vi "jojo_0822_copy.vi"() -> ()   [LabVIEW 2021]
uses:
  <vilib>/numeric/Random Number (Range) U64.vi
  <vilib>/numeric/sub_Random U32.vi
panel:
  out "Mixed Signal Graph 10":T1(graph)
  out "Mixed Signal Graph 9":T2(graph)
  out "Mixed Signal Graph 8":cluster{"Present (s)":dbl, "number":u64}[](graph)
  out "Mixed Signal Graph 7":cluster{"Present (s)":dbl, "number":u64}[](graph)
  out "Mixed Signal Graph 6":cluster{"Present (s)":dbl, "number":u64}[](graph)
  in  "Press to open Sub VI":bool
  in  "Update, Create, or Index File":string(combo)
  in  "File Name (include extension)":string
  out "error out":errorcluster
  out "Mixed Signal Graph 1":cluster{"Present (s)":dbl, "number":u64}[](graph)
  out "Mixed Signal Graph 2":cluster{"Present (s)":dbl, "number":u64}[](graph)
  out "Mixed Signal Graph 3":cluster{"Present (s)":dbl, "number":u64}[](graph)
  out "Mixed Signal Graph 5":T1(graph)
  out "Mixed Signal Graph 4":T2(graph)
  out "Elapsed Time (s)":dbl format="%<%H:%M:%S\n%y/%m/%d>T"
  out "millisecond timer value":u32
  in  "stop":bool
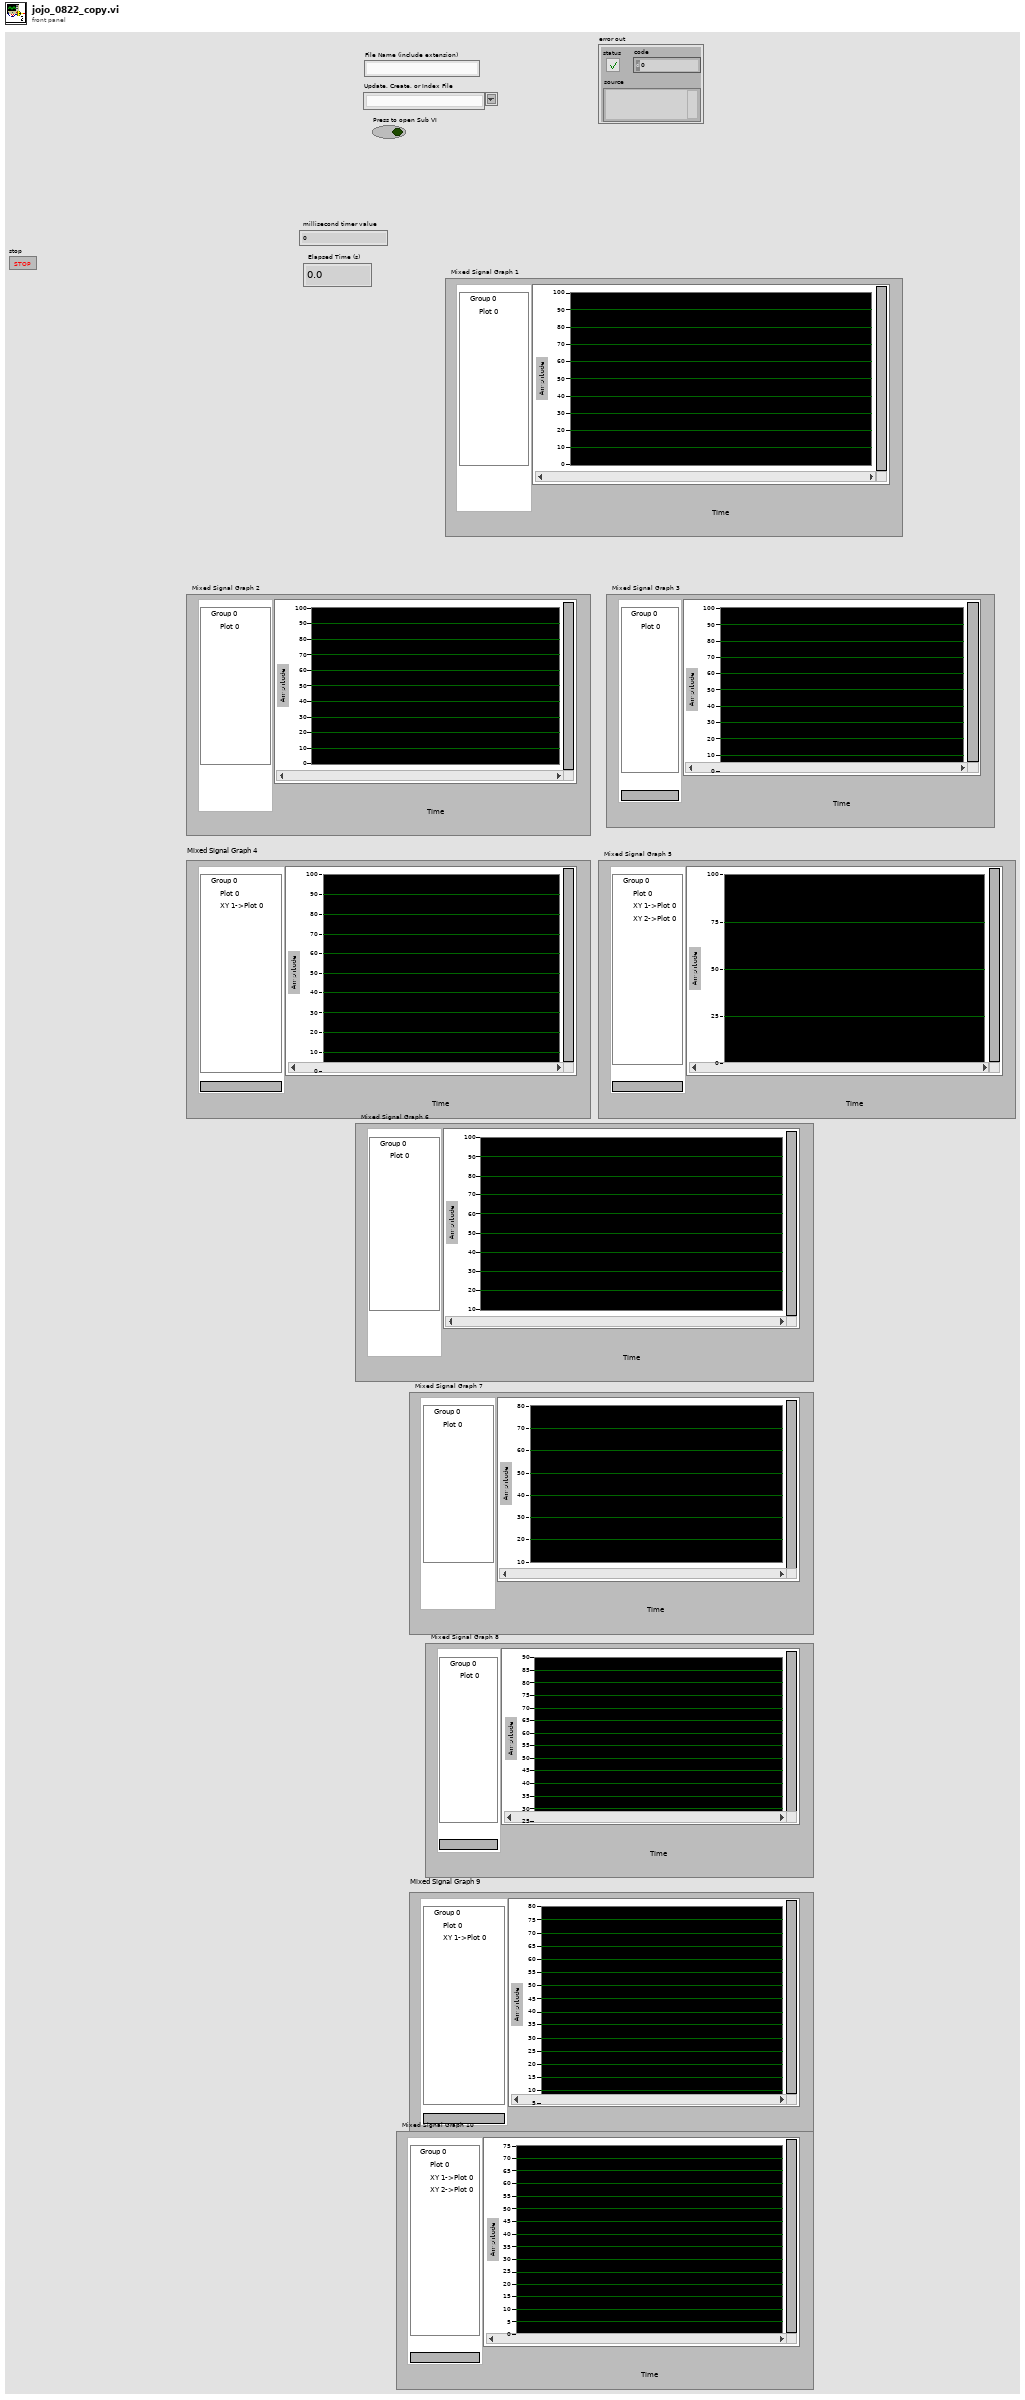
[diagram p1: front panel]
types:
  T1 = cluster{cluster{"Present (s)":dbl, "number":u64}[], cluster{"Present (s)":dbl, "number":u64}[], cluster{"Present (s)":dbl, "number":u64}[]}
  T2 = cluster{cluster{"Present (s)":dbl, "number":u64}[], cluster{"Present (s)":dbl, "number":u64}[]}
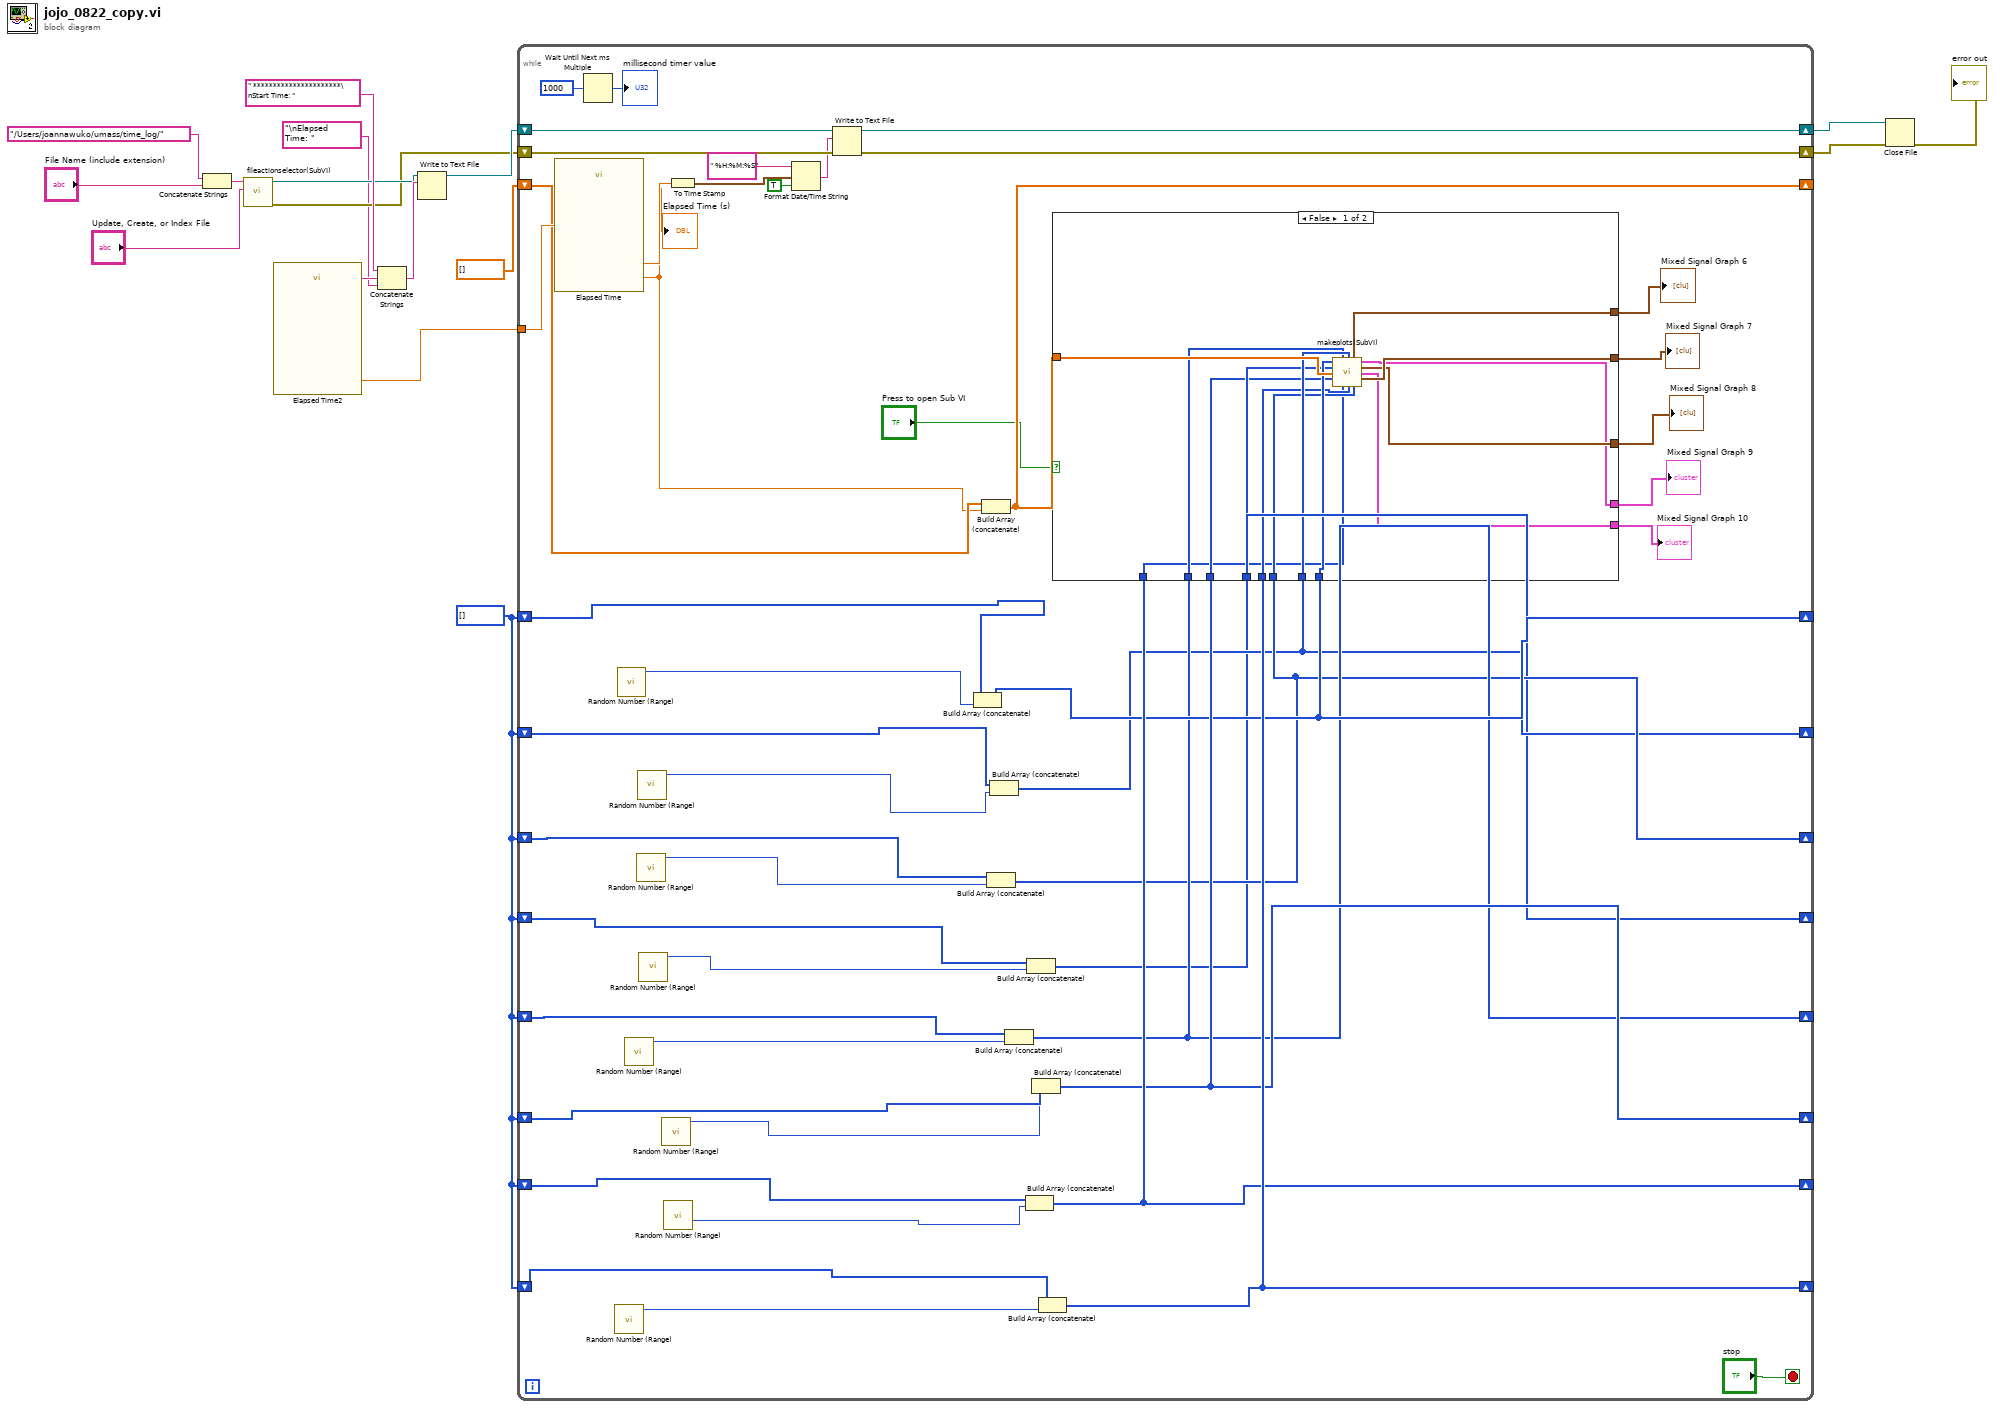
[diagram p0: block diagram]
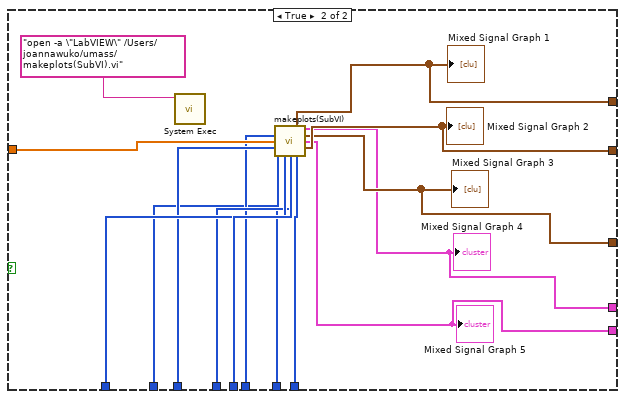
[diagram p2: hidden frame]
diagram:
  w15 = u64[] []
  n1 = Concatenate Strings("/Users/joannawuko/umass/time_log/" ("string"), "File Name (include extension)") -> (w3:string)
  n2 = call "fileactionselector(SubVI).vi"("Choose Update, Create, or Index File"="Update, Create, or Index File", "String"=w3) -> ("error out"=w4:errorcluster, "Byte Stream File out"=w5:refnum<file>)  [unwired: 8 in]
  n3 = call "Elapsed Time2"() -> ("Start Time Text"=w10:string, "Present (s)"=w17:dbl)  [unwired: 12 in, 6 out]
  n4 = Concatenate Strings(" **********************\nStart Time: ", w10, "\nElapsed Time: ") -> (w9:string)
  n5 = Write to Text File(file (use dialog)=w5, text=w9) -> (refnum out=w8:refnum<file>)  [unwired: 2 in, 2 out]
  n6 = while {
    shift-right: [w20] -> _
    shift-left: w15 -> [w38]
    shift-right: [w28] -> _
    shift-left: w15 -> [w36]
    shift-right: [w19] -> _
    shift-left: w15 -> [w34]
    shift-right: [w18] -> _
    shift-left: w15 -> [w40]
    shift-right: [w27] -> _
    shift-left: w15 -> [w42]
    shift-right: [w29] -> _
    shift-left: w15 -> [w44]
    shift-right: [w30] -> _
    shift-left: w15 -> [w46]
    shift-right: [w31] -> _
    shift-left: w15 -> [w48]
    tunnel: w17 -> [w60]
    shift-right: [w32] -> _
    shift-left: dbl[] [] -> [w50]
    shift-right: [w59] -> w14
    shift-left: w8 -> [w56]
    shift-right: [w58] -> w13
    shift-left: w4 -> [w57]
    stop <- "stop" stop-if-true
    n7 = call "Elapsed Time"("Set Start Time (s)"=w60) -> ("Present (s)"=w49:dbl, "Elapsed Time (s)"=w55:dbl)  [unwired: 11 in, 6 out]
    "Elapsed Time (s)" <- w49
    n8 = Wait Until Next ms Multiple(millisecond multiple=u32 1000) -> (millisecond timer value=→"millisecond timer value":u32)
    n9 = call-poly <vilib>:"Random Number (Range).vi"() -> ("number"=w47:u64)  [unwired: 11 in]
    n10 = call-poly <vilib>:"Random Number (Range).vi"() -> ("number"=w35:u64)  [unwired: 11 in]
    n11 = call-poly <vilib>:"Random Number (Range).vi"() -> ("number"=w41:u64)  [unwired: 11 in]
    n12 = call-poly <vilib>:"Random Number (Range).vi"() -> ("number"=w37:u64)  [unwired: 11 in]
    n13 = call-poly <vilib>:"Random Number (Range).vi"() -> ("number"=w33:u64)  [unwired: 11 in]
    n14 = call-poly <vilib>:"Random Number (Range).vi"() -> ("number"=w39:u64)  [unwired: 11 in]
    n15 = call-poly <vilib>:"Random Number (Range).vi"() -> ("number"=w43:u64)  [unwired: 11 in]
    n16 = call-poly <vilib>:"Random Number (Range).vi"() -> ("number"=w45:u64)  [unwired: 11 in]
    n17 = To Time Stamp(1:w55) -> (0:w51:timestamp)
    n18 = Format Date/Time String(time format string (%c)=" %H:%M:%S", seconds (now)=w51, UTC format=TRUE) -> (date/time string=w54:string)
    n19 = Write to Text File(file (use dialog)=w56, text=w54, error in=w57) -> (refnum out=w59:refnum<file>, error out=w58:errorcluster)  [unwired: 1 in, 1 out]
    n20 = Build Array (concatenate)(w36, w35) -> (w28:u64[])
    n21 = Build Array (concatenate)(w50, w49) -> (w32:dbl[])
    n22 = Build Array (concatenate)(w38, w37) -> (w20:u64[])
    n23 = Build Array (concatenate)(w34, w33) -> (w19:u64[])
    n24 = Build Array (concatenate)(w42, w41) -> (w27:u64[])
    n25 = Build Array (concatenate)(w46, w45) -> (w30:u64[])
    n26 = Build Array (concatenate)(w40, w39) -> (w18:u64[])
    n27 = Build Array (concatenate)(w44, w43) -> (w29:u64[])
    n28 = Build Array (concatenate)(w48, w47) -> (w31:u64[])
    n29 = case shown="False" "Press to open Sub VI" {
      tunnel: w32 -> [w72 w92]
      tunnel: w31 -> [w67 w91]
      tunnel: w30 -> [w64 w90]
      tunnel: w29 -> [w66 w89]
      tunnel: w18 -> [w68 w88]
      tunnel: w20 -> [w69 w87]
      tunnel: w28 -> [w71 w86]
      tunnel: w19 -> [w70 w85]
      tunnel: w27 -> [w65 w84]
      tunnel: [w77 w82] -> w25
      tunnel: [w76 w81] -> w24
      tunnel: [w75 w80] -> w23
      tunnel: [w74 w79] -> w22
      tunnel: [w73 w78] -> w21
      frame False {
        n30 = call "makeplots(SubVI).vi"("Array"=w71, "Array 5"=w65, "Array 2"=w70, "Array 4"=w68, "Array 9"=w72, "Array 6"=w66, "Array 7"=w64, "Array 8"=w67, "Array 3"=w69) -> ("Mixed Signal Graph 1"=w77:cluster{"Present (s)":dbl, "number":u64}[], "Mixed Signal Graph 4"=w74:T2, "Mixed Signal Graph 3"=w75:cluster{"Present (s)":dbl, "number":u64}[], "Mixed Signal Graph 5"=w73:T1, "Mixed Signal Graph 2"=w76:cluster{"Present (s)":dbl, "number":u64}[])  [unwired: 2 in]
      }
      frame True {
        n31 = call <vilib>:"System Exec.vi"("command line"="open -a \"LabVIEW\" /Users/joannawuko/umass/makeplots(SubVI).vi") -> ()  [unwired: 7 in, 4 out]
        n32 = call "makeplots(SubVI).vi"("Array"=w84, "Array 5"=w88, "Array 2"=w85, "Array 4"=w87, "Array 9"=w92, "Array 6"=w89, "Array 7"=w90, "Array 8"=w91, "Array 3"=w86) -> ("Mixed Signal Graph 1"=w82:cluster{"Present (s)":dbl, "number":u64}[], "Mixed Signal Graph 4"=w79:T2, "Mixed Signal Graph 3"=w80:cluster{"Present (s)":dbl, "number":u64}[], "Mixed Signal Graph 5"=w78:T1, "Mixed Signal Graph 2"=w81:cluster{"Present (s)":dbl, "number":u64}[])  [unwired: 2 in]
        "Mixed Signal Graph 1" <- w82
        "Mixed Signal Graph 2" <- w81
        "Mixed Signal Graph 3" <- w80
        "Mixed Signal Graph 4" <- w79
        "Mixed Signal Graph 5" <- w78
      }
    }
    "Mixed Signal Graph 6" <- w25
    "Mixed Signal Graph 7" <- w24
    "Mixed Signal Graph 8" <- w23
    "Mixed Signal Graph 9" <- w22
    "Mixed Signal Graph 10" <- w21
  }
  n33 = Close File(refnum=w14, error in=w13) -> (error out=→"error out":errorcluster)  [unwired: 1 out]
